vi "Week_4_4.1_Example-3.vi"() -> ()   [LabVIEW 2015]
panel:
  in  "stop":bool
  out "Waveform Graph":dynamicdata(graph)
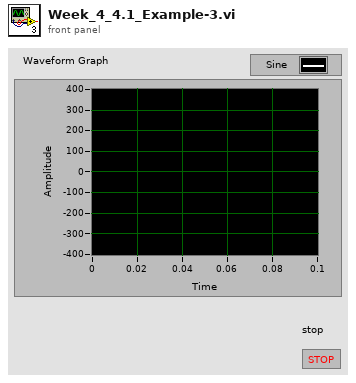
[diagram p1: front panel]
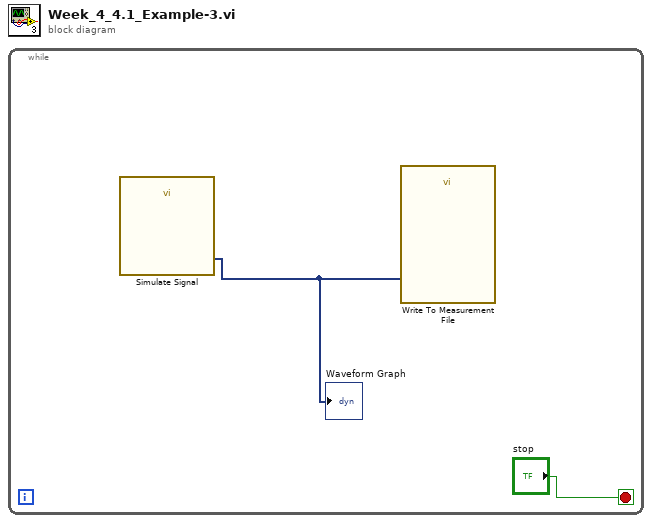
[diagram p0: block diagram]
diagram:
  n1 = while {
    stop <- "stop" stop-if-true
    n2 = call "Simulate Signal"() -> ("Sine"=w2:dynamicdata)  [unwired: 14 in, 1 out]
    "Waveform Graph" <- w2
    n3 = call "Write To Measurement File"("Signals"=w2) -> ()  [unwired: 16 in, 3 out]
  }
